vi "Identify Action.vi"(8 "error in (no error)":errorcluster, 10 "Item Tag":string) -> (0 "error out":errorcluster, 3 "RCM_Actions out":refnum<class "RCM_Actions.lvclass">)   [LabVIEW 2016, in "Assert API Components.lvlib" / "Assert Display.lvlib" / "Main Display.lvlib" / "RCM_Actions.lvclass"]
uses:
  RCM_Actions.lvclass
  Change Column Header/Change Column Header.lvclass
  C:/Users/ukhornp/Documents/Work/Projects/actor_assert_api/Core/Main Display/Right Click Menu Actions/RCM_Actions.lvclass
  Change Column Header/Change Column Header.lvclass/Change Column Header.ctl
  Change Failure Action/Change Failure Action.lvclass
  Change Failure Action/Change Failure Action.lvclass/Change Failure Action.ctl
  Show Assert/Show Assert.lvclass
  Show Assert/Show Assert.lvclass/Show Assert.ctl
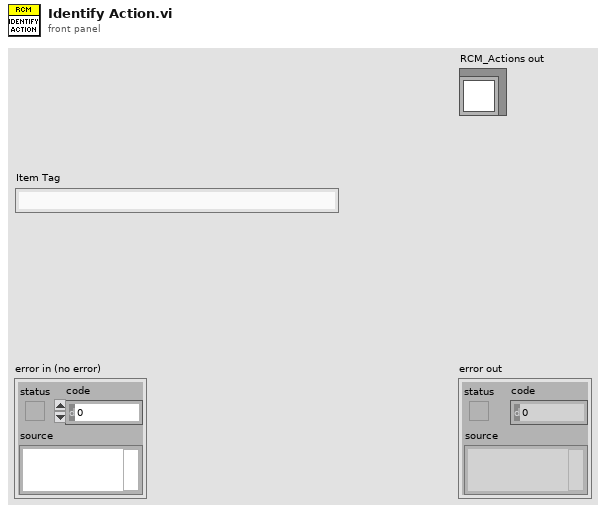
[diagram p1: front panel]
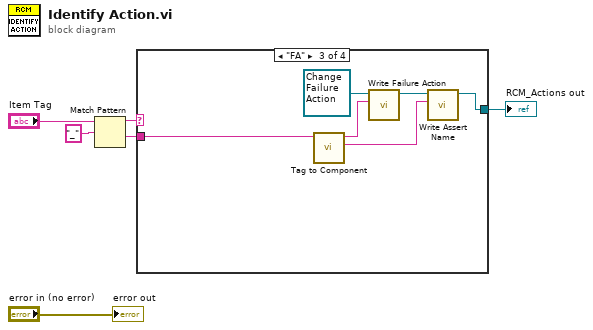
[diagram p0: block diagram]
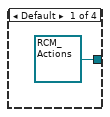
[diagram p2: hidden frame]
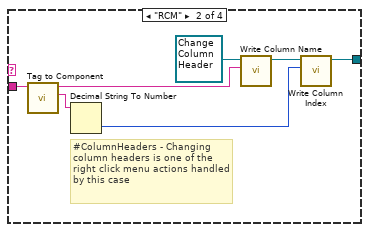
[diagram p3: hidden frame]
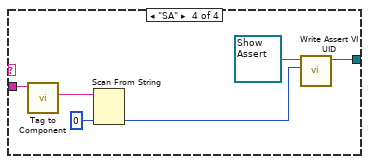
[diagram p4: hidden frame]
diagram:
  n1 = Match Pattern(string="Item Tag", regular expression="_") -> (before substring=w3:string, after substring=w4:string)  [unwired: 1 in, 2 out]
  n2 = case shown="\"FA\"" w3 {
    tunnel: w4 -> [_ w13 w20 w26]
    tunnel: [refnum<class "RCM_Actions.lvclass"> refnum ("RCM_Actions out") w10 w15 w25] -> w2
    frame Default {
    }
    frame "RCM" {
      # "#ColumnHeaders - Changing column headers is one of the right click menu actions handled by this case"
      n3 = call "Tag to Component.vi"("Item Tag in"=w13) -> ("Component Value"=w14:string, "Component Name"=w9:string)  [unwired: 9 in]
      n4 = Decimal String To Number(string=w14) -> (number=w8:i32)  [unwired: 2 in, 1 out]
      n5 = call "Write Column Name.vi"("Column Name"=w9, "Change Column Header in"=refnum<class "Change Column Header.lvclass"> refnum ("Assert API Components.lvlib:Assert Display.lvlib:Main Display.lvlib:Change Column Header.lvclass")) -> ("Change Column Header out"=w11:refnum<class "Change Column Header.lvclass">)  [unwired: 9 in]
      n6 = call "Write Column Index.vi"("Column Index"=w8, "Change Column Header in"=w11) -> ("Change Column Header out"=w10:refnum<class "Change Column Header.lvclass">)  [unwired: 9 in]
    }
    frame "FA" {
      n7 = call "Tag to Component.vi"("Item Tag in"=w20) -> ("Component Value"=w19:string, "Component Name"=w18:string)  [unwired: 9 in]
      n8 = call "Write Failure Action.vi"("Failure Action"=w18, "Change Failure Action in"=refnum<class "Change Failure Action.lvclass"> refnum ("Assert API Components.lvlib:Assert Display.lvlib:Main Display.lvlib:Change Failure Action.lvclass")) -> ("Change Failure Action out"=w16:refnum<class "Change Failure Action.lvclass">)  [unwired: 9 in]
      n9 = call "Write Assert Name.vi"("Assert UID"=w19, "Change Failure Action in"=w16) -> ("Change Failure Action out"=w15:refnum<class "Change Failure Action.lvclass">)  [unwired: 9 in]
    }
    frame "SA" {
      n10 = call "Tag to Component.vi"("Item Tag in"=w26) -> ("Component Value"=w22:string)  [unwired: 9 in, 1 out]
      n11 = Scan From String(input string=w22, default 1=0 ("Assert VI UID")) -> (output 1=w21:i32)  [unwired: 3 in, 3 out]
      n12 = call "Write Assert VI UID.vi"("Assert VI UID"=w21, "Show Assert in"=refnum<class "Show Assert.lvclass"> refnum ("Assert API Components.lvlib:Assert Display.lvlib:Main Display.lvlib:Show Assert.lvclass")) -> ("Show Assert out"=w25:refnum<class "Show Assert.lvclass">)  [unwired: 9 in]
    }
  }
  "RCM_Actions out" <- w2
  "error out" <- "error in (no error)"
